vi "diode curve tracer -- step V_D.vi"() -> ()   [LabVIEW 2016]
doc: "Diode curve tracer for the NI myDAQ. Requires a 100-ohm resistor and an operation amplifier (op amp)."
uses:
  <vilib>/Analysis/1siggen.llb/Ramp Pattern by Delta.vi
  <vilib>/Analysis/NI_AALBase.lvlib
panel:
  in  "Tab Control":T1(tab)
  in  "RD [ohm]":dbl=100.0
  in  "V_D start [V]":dbl
  in  "V_D stop [V]":dbl=0.8
  in  "V_D step [V]":dbl=0.05
  in  "step time [ms]":u32=100
  out "XY Graph":cluster{dbl, dbl}[](graph)
  out "Over\nCurrent":bool
  out "Progress":u8(slide)=100 scale=0.0..100.0
  # "Diode Curve Tracer"
  # "Instructions:\n\n- Establish the NI myDAQ connections to the diode, diode resistor,\n     and op amp as shown on the \"Connection Diagram\" tab\n\n- Select the diode resistor and measure its value with the\n      myDAQ ohmmeter\n\n- Enter the measured diode resistance as \"RD\" in ohms\n\n- Enter the start, stop, and step values for the diode voltage \"V_D\"\n\n- Click the run button or type Ctrl+R to perform the measurement\n\n- The \"Over Current\" indicator lights up when the opamp is unable\n      to supply the needed current to attain the desired diode voltage\n\n- Adjust the \"step time\" to speed up or slow down the measurement\n\n- Right-click on the graph and choose \"Export\" to save the datapoints\n     to a file or to create a plot image to be pasted into a document"
  # "Theory of Operation:\n\n- The desired diode voltage appears on Analog Output 0 (AO0)\n\n- The opamp circuit uses negative feedback to adjust the diode\n      resistor voltage (left side) to make the actual diode voltage match\n      the desired voltage. When the op amp current output current is\n      insufficient to make this happen, the actual diode voltage falls\n      short of the intended voltage.\n\n- The actual diode voltage V_D is measured by Analog Input 1 (AI1)\n\n- The resistor voltage measured by Analog Input 0 (AI0) divided by\n      the measured value of the diode resistor RD yields the diodecurrent I_D"
  # "- Any typical op amp should work fine.\n\n- 100 ohms (brown-black-brown color code) works well for RD."
  # "Plot Axes:\n\n- Right-click on the plot axis to disable \"Auto Scaling\" which is\n     enabled by default\n\n- When \"Auto Scaling\" is disabled, double-click the plot axis limits\n      and enter new values as needed\n\n- Right-click on the plot axis and choose \"Mapping\" to select\n     between logarithmic and linear modes"
  # "Cursors:\n\n- Click and drag the vertical cursor line on the far left side of the plot;\n     read the cursor value in the panel below the graph; the active\n     cursor indictor is highlighted in yellow.\n\n- Click the right and left buttons of the diamond to step the cursors\n     from one point to the next.\n\n- Click the cursor icon to activate both cursors, and then click the\n     diamond buttons to move both cursors at the same time."
  # "Exporting Measurement Data:\n\n- Right-click on the graph and choose \"Export\" to save the measurements\n     to a file or to create a plot image to be pasted into a document."
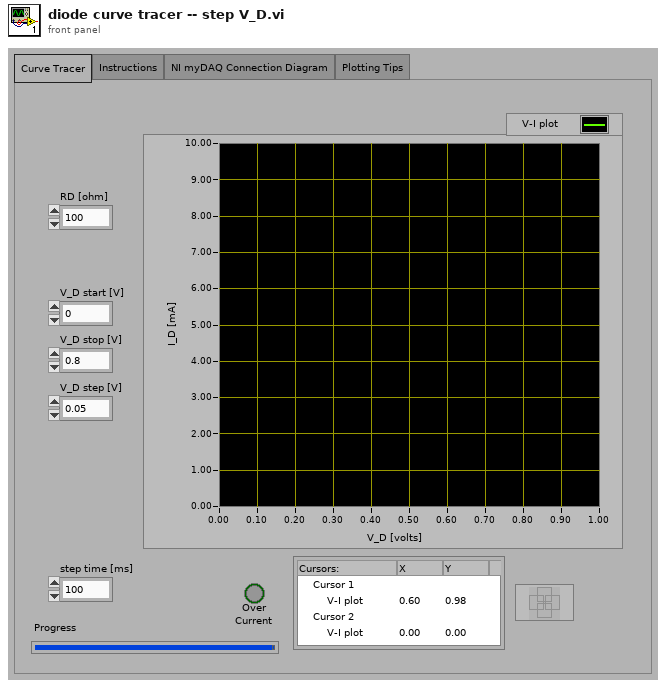
[diagram p1: front panel]
types:
  T1 = enum32{"Curve Tracer", "Instructions", "NI myDAQ Connection Diagram", "Plotting Tips"}
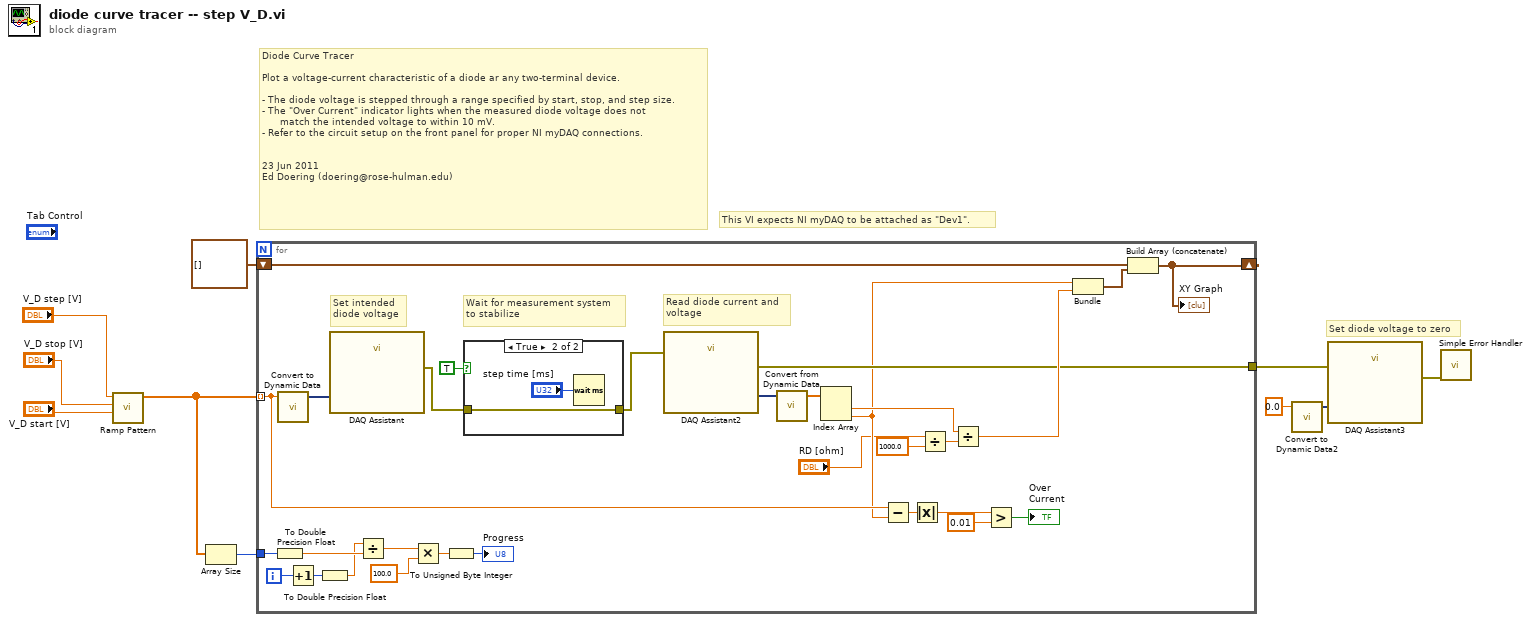
[diagram p0: block diagram]
diagram:
  # "This VI expects NI myDAQ to be attached as \"Dev1\"."
  # "Diode Curve Tracer\n\nPlot a voltage-current characteristic of a diode ar any two-terminal device.\n\n- The diode voltage is stepped through a range specified by start, stop, and step size.\n- The \"Over Current\" indicator lights when the measured diode voltage does not\n      match the intended voltage to within 10 mV.\n- Refer to the circuit setup on the front panel for proper NI myDAQ connections.\n\n\n23 Jun 2011\nEd Doering (doering@rose-hulman.edu)"
  # "Set diode voltage to zero"
  n1 = call-poly <vilib>:"Ramp Pattern.vi"("start"="V_D start [V]", "end"="V_D stop [V]", "delta"="V_D step [V]") -> ("Ramp Pattern"=w3:dbl[])  [unwired: 6 in, 2 out]
  n2 = Array Size(array=w3) -> (size(s)=w2:i32)
  n3 = for {
    tunnel: w3 -> [w28] mode=indexing
    shift-right: [w30] -> _
    shift-left: cluster{dbl, dbl}[] [] -> [w31]
    tunnel: [w29] -> w6
    tunnel: w2 -> [w20]
    i -> [w16]
    # "Wait for measurement system\nto stabilize"
    # "Read diode current and\nvoltage"
    # "Set intended\ndiode voltage"
    n4 = To Double Precision Float(number=w20) -> (double precision float=w19:dbl)
    n5 = call "Convert to Dynamic Data"("Double"=w28) -> ("Dynamic Data Type"=w40:dynamicdata)  [unwired: 3 in]
    n6 = Increment(x=w16) -> (x+1=w15:i32)
    n7 = To Double Precision Float(number=w15) -> (double precision float=w14:dbl)
    n8 = call "DAQ Assistant"("data"=w40) -> ("error out"=w36:errorcluster)  [unwired: 17 in, 1 out]
    n9 = Divide(x=w14, y=w19) -> (x/y=w22:dbl)
    n10 = Multiply(x=w22, y=100.0) -> (x*y=w17:dbl)
    n11 = To Unsigned Byte Integer(number=w17) -> (unsigned 8bit integer=→"Progress":u8)
    n12 = case shown="True" TRUE {
      tunnel: w36 -> [_ w41]
      tunnel: [_ w41] -> w35
      frame False {
      }
      frame True {
        n13 = Wait (ms)(milliseconds to wait="step time [ms]") -> ()  [unwired: 1 out]
      }
    }
    n14 = call "DAQ Assistant2"("error in"=w35) -> ("data"=w39:dynamicdata, "error out"=w29:errorcluster)  [unwired: 16 in, 1 out]
    n15 = call "Convert from Dynamic Data"("Dynamic Data Type"=w39) -> ("Array"=w38:dbl[])  [unwired: 3 in]
    n16 = Index Array(array=w38) -> (element #1=w37:dbl, element #2=w27:dbl)  [unwired: 2 in]
    n17 = Subtract(x=w28, y=w27) -> (x-y=w26:dbl)
    n18 = Absolute Value(x=w26) -> (abs(x)=w25:dbl)
    n19 = Divide(x="RD [ohm]", y=1000.0) -> (x/y=w13:dbl)
    n20 = Divide(x=w37, y=w13) -> (x/y=w33:dbl)
    n21 = Greater?(x=w25, y=0.01) -> (0:→"Over\nCurrent":bool)
    n22 = Bundle(w27, w33) -> (w32:cluster{dbl, dbl})  [unwired: 1 in]
    n23 = Build Array (concatenate)(w31, w32) -> (w30:cluster{dbl, dbl}[])
    "XY Graph" <- w30
  }
  n24 = call "Convert to Dynamic Data2"("Double"=0.0) -> ("Dynamic Data Type"=w5:dynamicdata)  [unwired: 3 in]
  n25 = call "DAQ Assistant3"("data"=w5, "error in"=w6) -> ("error out"=w1:errorcluster)  [unwired: 16 in, 1 out]
  n26 = call <vilib>:"Simple Error Handler.vi"("error in (no error)"=w1) -> ()  [unwired: 4 in, 5 out]
